vi "数字输入_软件按需单点(线).vi"() -> ()   [LabVIEW 2013]
doc: "This example demonstrates how to read values from multi digital input lines(channels)."
uses:
  <userlib>/ArtDAQ/_SubVI/ArtDAQ_CreateDIChan.vi
  <userlib>/ArtDAQ/_SubVI/ArtDAQ_Read Digital Bool 1Chan 1Samp.vi
panel:
  out "?":bool
  out "错误输出":errorcluster
  in  "?":bool
  in  "超时(ms)":u32=10
  in  "线通道":string="Dev1/port0/line7"
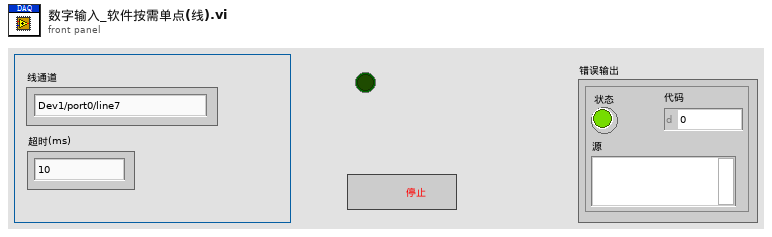
[diagram p1: front panel]
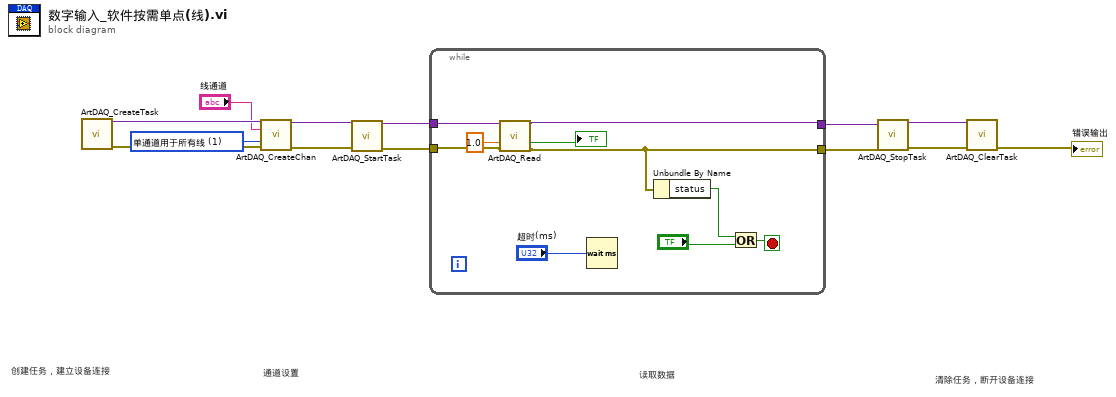
[diagram p0: block diagram]
diagram:
  w5 = 1 items=["单通道用于单条线", "单通道用于所有线"] ("Line Grouping")
  # "清除任务，断开设备连接"
  # "读取数据"
  # "通道设置"
  # "创建任务，建立设备连接"
  n1 = call <userlib>:"ArtDAQ_CreateTask.vi"() -> ("任务句柄"=w4:variant, "错误输出"=w3:errorcluster)  [unwired: 14 in]
  n2 = call-poly <userlib>:"ArtDAQ_CreateChan.vi"("任务句柄"=w4, "线"="线通道", "线分组"=w5, "错误输入"=w3) -> ("任务句柄"=w13:variant, "错误输出"=w12:errorcluster)  [unwired: 10 in]
  n3 = call <userlib>:"ArtDAQ_StartTask.vi"("任务句柄"=w13, "错误输入"=w12) -> ("任务句柄"=w11:variant, "错误输出"=w10:errorcluster)  [unwired: 12 in]
  n4 = while {
    tunnel: w11 -> [w19]
    tunnel: w10 -> [w17]
    tunnel: [w18] -> w9
    tunnel: [w16] -> w8
    stop <- w21 stop-if-true
    n5 = call-poly <userlib>:"ArtDAQ_Read.vi"("任务句柄"=w19, "超时s"=1.0 ("Timeout"), "错误输入"=w17) -> ("任务句柄"=w18:variant, "数据"=→"?":bool, "错误输出"=w16:errorcluster)  [unwired: 10 in]
    n6 = Wait (ms)(milliseconds to wait="超时(ms)") -> ()  [unwired: 1 out]
    n7 = Unbundle By Name(w16) -> ("status"=w22:bool)
    n8 = Or(x=w22, y="?") -> (x .or. y?=w21:bool)
  }
  n9 = call <userlib>:"ArtDAQ_StopTask.vi"("任务句柄"=w9, "错误输入"=w8) -> ("任务句柄"=w6:variant, "错误输出"=w7:errorcluster)  [unwired: 12 in]
  n10 = call <userlib>:"ArtDAQ_ClearTask.vi"("任务句柄"=w6, "错误输入"=w7) -> ("错误输出"=→"错误输出":errorcluster)  [unwired: 13 in]
